vi "keccak.ip.fifo.control.vi"(10 "FIFO.inputs":T2, 11 "Reset":bool) -> (3 "FIFO.outputs":T1)   [LabVIEW 2021]
uses:
  Users/johns/OneDrive/Documents/LabVIEW Data/Untitled Project 2/CLIP/keccak.variables.ctl
  Users/johns/OneDrive/Documents/LabVIEW Data/Untitled Project 2/CLIP/keccak.states.ctl
  <vilib>/rvi/Emulation/niFpgaEmulationIsFPGAContextNoSignature.vi
  <vilib>/rvi/Emulation/niFpgaSctlEmulationGetInTimedLoop.vi
  <vilib>/rvi/errors/niFpgaSetErrorForExecOnDevCompSimple.vi
  <vilib>/rvi/eio/common/nirviEmuReportErrorAndStop.vi
  <vilib>/rvi/DataTransferAndStorage/Container/Common/niFpgaContainerGetUniqueNameForEmu.vi
  <vilib>/rvi/FIFO/Fifo_Resource/nirvififoEmulationSetSize.vi
  <vilib>/rvi/FIFO/Fifo_Resource/nirviFifoEmulationQueueMgr.vi
  <instcachedir>/0/nirviFifoEmulationQueueMgr_E5CAEC123FF24DC58D834DCA3CDAA9B5.lvgen/nirviFifoEmulationQueueMgr_E5CAEC123FF24DC58D834DCA3CDAA9B5_000.vi
  <vilib>/Utility/error.llb/Clear Errors.vi
  <vilib>/rvi/FIFO/Fifo_Resource/nirvififoEmulationCreateLock.vi
  <vilib>/rvi/Emulation/niFpgaProcessEmulError.vi
  <vilib>/rvi/FIFO/Fifo_Resource/nirvififoEmulationObtainLock.vi
  <vilib>/rvi/FIFO/Fifo_Resource/nirvififoEmulationReleaseLock.vi
  <vilib>/rvi/occurrence/nirviWaitOnOccurrenceBase.vi
  <vilib>/rvi/errors/nirviReportUnexpectedCaseInternalError.vi
  <vilib>/rvi/errors/nirviReportUnexpectedCaseInternalError (U32).vi
  <vilib>/rvi/FIFO/Fifo_Resource/nirvififoEmulationDetermineInputValidOut.vi
  <vilib>/rvi/DataTransferAndStorage/Container/XNode/niFpgaContainer.xnode
  <vilib>/rvi/FIFO/Fifo_Resource/nirvififoEmulationRead.vi
  <vilib>/rvi/FIFO/Fifo_Resource/nirvififoEmulationWrite.vi
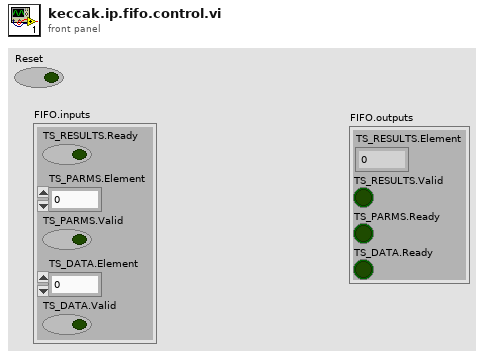
[diagram p1: front panel]
types:
  T1 = cluster{"TS_RESULTS.Element":u64, "TS_RESULTS.Valid":bool, "TS_PARMS.Ready":bool, "TS_DATA.Ready":bool}
  T2 = cluster{"TS_RESULTS.Ready":bool, "TS_PARMS.Element":u64, "TS_PARMS.Valid":bool, "TS_DATA.Element":u64, "TS_DATA.Valid":bool}
  T3 = typedef "keccak.variables.ctl" = cluster{"hash.input_size":u16, "hash.bits":u16, "state.next":T4, "state.after_next":T4, "read.i":u16, "read.block_i":u16, "hash.block_words":u16, "hash.block_size":u16, "keccak.i":u16, "state[25]":u64[], "HT_PARMS.Valid":bool, "HT_PARMS.Data":u64, "Read.HT_PARMS":bool, "HT_DATA.Valid":bool, "HT_DATA.Data":u64, "Read.HT_DATA":bool, "TH_RESULTS.Valid":bool, "TH_RESULTS.Data":u64, "TH_RESULTS.Ready":bool}
  T4 = typedef "keccak.states.ctl" = enum8{"Wait.for.Start", "Read.Blocks", "Read.Remainder", "Keccak", "Send.Result"}
  T5 = cluster{"Element":u64, bool, "Timed Out?":bool, "Ready for Input":bool}
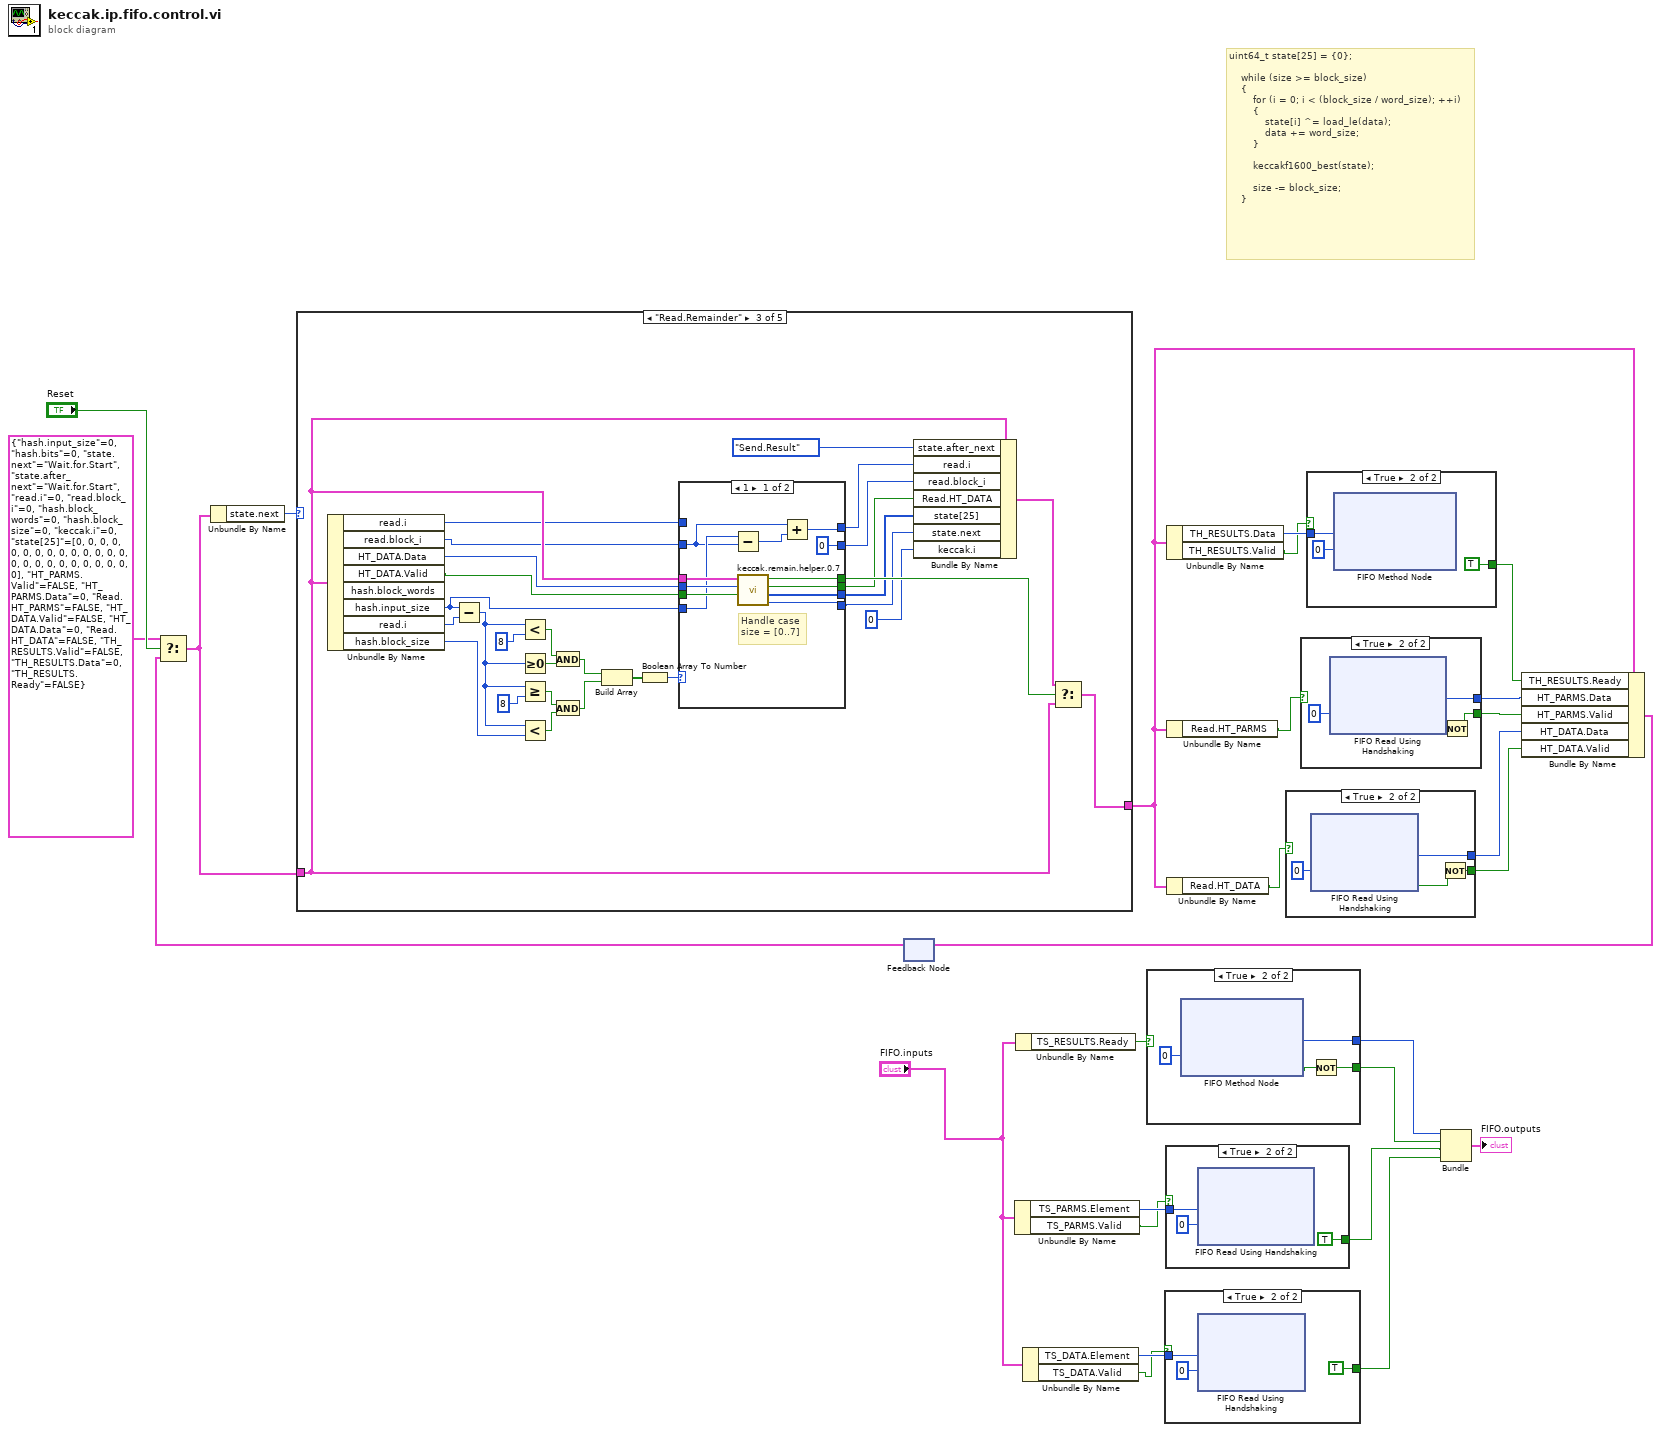
[diagram p0: block diagram]
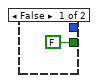
[diagram p2: hidden frame]
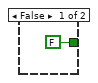
[diagram p3: hidden frame]
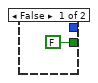
[diagram p4: hidden frame]
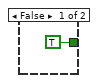
[diagram p5: hidden frame]
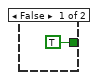
[diagram p6: hidden frame]
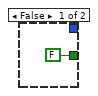
[diagram p7: hidden frame]
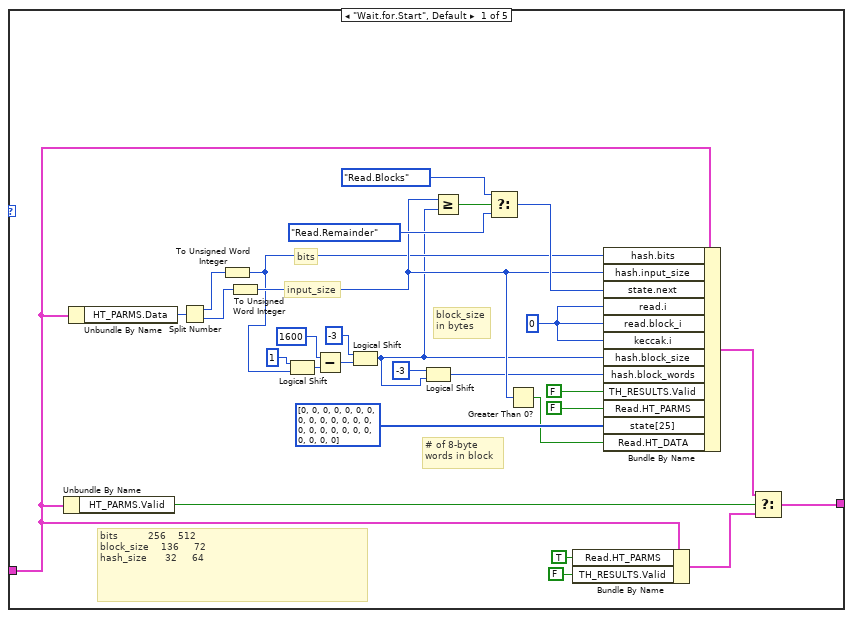
[diagram p8: hidden frame]
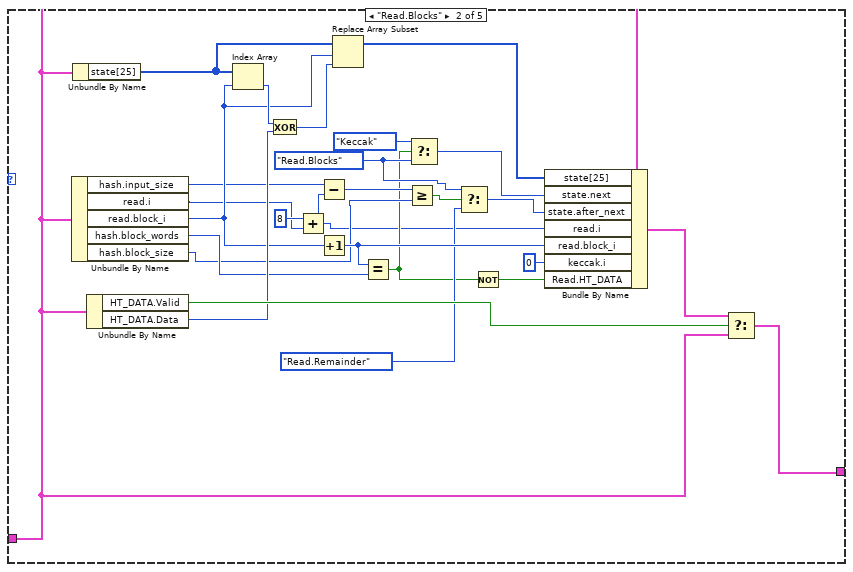
[diagram p9: hidden frame]
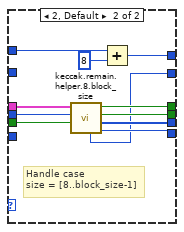
[diagram p10: hidden frame]
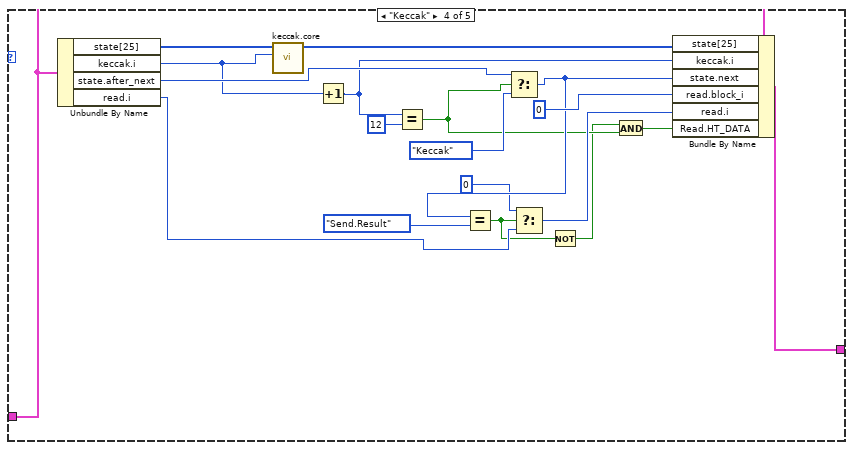
[diagram p11: hidden frame]
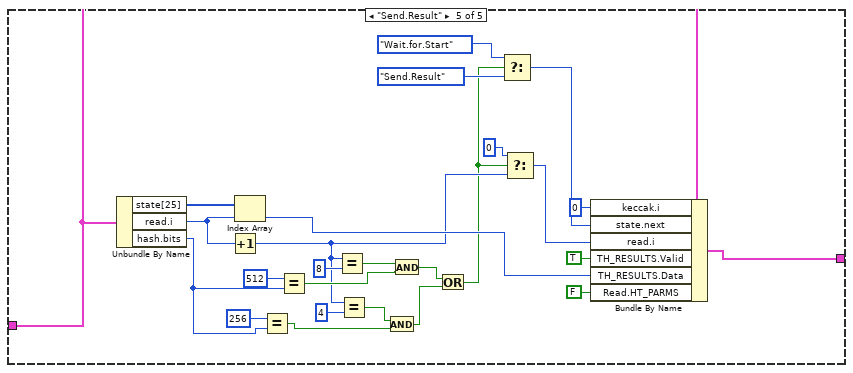
[diagram p12: hidden frame]
diagram:
  # "uint64_t state[25] = {0};\n\n    while (size >= block_size)\n    {\n        for (i = 0; i < (block_size / word_size); ++i)\n        {\n            state[i] ^= load_le(data);\n            data += word_size;\n        }\n\n        keccakf1600_best(state);\n\n        size -= block_size;\n    }"
  n1 = feedback #1() -> (w16:T3)  [unwired: 1 in]
  n2 = Select(t=T3 {"hash.input_size"=0, "hash.bits"=0, "state.next"=enum."Wait.for.Start", "state.after_next"=enum."Wait.for.Start", "read.i"=0, "read.block_i"=0, "hash.block_words"=0, "hash.block_size"=0, "keccak.i"=0, "state[25]"=[0, 0, 0, 0, 0, 0, 0, 0, 0, 0, 0, 0, 0, 0, 0, 0, 0, 0, 0, 0, 0, 0, 0, 0, 0], "HT_PARMS.Valid"=FALSE, "HT_PARMS.Data"=0, "Read.HT_PARMS"=FALSE, "HT_DATA.Valid"=FALSE, "HT_DATA.Data"=0, "Read.HT_DATA"=FALSE, "TH_RESULTS.Valid"=FALSE, "TH_RESULTS.Data"=0, "TH_RESULTS.Ready"=FALSE} ("Variables"), s="Reset", f=w16) -> (s? t:f=w15:T3)
  n3 = Unbundle By Name(w15) -> ("state.next"=w27:T4)
  n4 = case shown="\"Read.Remainder\"" w27 {
    tunnel: [w52 w82 w109 w152 w180] -> w22
    tunnel: w15 -> [w47 w81 w105 w153 w179]
    frame "Wait.for.Start", Default {
      w37 = u16 0 ("read.i")
      # "# of 8-byte\nwords in block"
      # "block_size\nin bytes"
      # "bits"
      # "input_size"
      # "bits          256    512\nblock_size    136     72\nhash_size      32     64"
      n5 = Unbundle By Name(w47) -> ("HT_PARMS.Valid"=w51:bool)
      n6 = Unbundle By Name(w47) -> ("HT_PARMS.Data"=w56:u64)
      n7 = Split Number(x=w56) -> (hi(x)=w55:u32, lo(x)=w54:u32)
      n8 = To Unsigned Word Integer(number=w55) -> (unsigned 16bit integer=w29:u16)
      n9 = To Unsigned Word Integer(number=w54) -> (unsigned 16bit integer=w39:u16)
      n10 = Logical Shift(y=i16 1, x=w29) -> (x << y=w34:u16)
      n11 = Subtract(x=u16 1600, y=w34) -> (x-y=w33:u16)
      n12 = Logical Shift(y=i16 -3, x=w33) -> (x << y=w28:u16)
      n13 = Logical Shift(y=i16 -3, x=w28) -> (x << y=w30:u16)
      n14 = Greater Or Equal?(x=w39, y=w28) -> (x >= y?=w43:bool)
      n15 = Select(t=keccak.states."Read.Blocks" ("state.next"), s=w43, f=keccak.states."Read.Remainder" ("state.next")) -> (s? t:f=w41:T4)
      n16 = Greater Than 0?(x=w39) -> (x > 0?=w38:bool)
      n17 = Bundle By Name(cluster=w47, "Read.HT_PARMS"=TRUE, "TH_RESULTS.Valid"=FALSE) -> (w48:T3)
      n18 = Bundle By Name(cluster=w47, "hash.bits"=w29, "hash.input_size"=w39, "state.next"=w41, "read.i"=w37, "read.block_i"=w37, "keccak.i"=w37, "hash.block_size"=w28, "hash.block_words"=w30, "TH_RESULTS.Valid"=FALSE, "Read.HT_PARMS"=FALSE, "state[25]"=u64[] [0, 0, 0, 0, 0, 0, 0, 0, 0, 0, 0, 0, 0, 0, 0, 0, 0, 0, 0, 0, 0, 0, 0, 0, 0] ("state[24]"), "Read.HT_DATA"=w38) -> (w53:T3)
      n19 = Select(t=w53, s=w51, f=w48) -> (s? t:f=w52:T3)
    }
    frame "Read.Blocks" {
      w62 = keccak.states."Read.Blocks" ("state.next")
      n20 = Unbundle By Name(w81) -> ("hash.input_size"=w67:u16, "read.i"=w66:u16, "read.block_i"=w75:u16, "hash.block_words"=w71:u16, "hash.block_size"=w63:u16)
      n21 = Unbundle By Name(w81) -> ("state[25]"=w79:u64[])
      n22 = Unbundle By Name(w81) -> ("HT_DATA.Valid"=w80:bool, "HT_DATA.Data"=w76:u64)
      n23 = Index Array(array=w79, index=w75) -> (element=w78:u64)
      n24 = Exclusive Or(1:w76, 2:w78) -> (0:w77:u64)
      n25 = Add(x=u16 8, y=w66) -> (x+y=w57:u16)
      n26 = Subtract(x=w67, y=w57) -> (x-y=w64:u16)
      n27 = Increment(x=w75) -> (x+1=w72:u16)
      n28 = Replace Array Subset(array=w79, new element=w77, index=w75) -> (w68:u64[])
      n29 = Equal?(x=w72, y=w71) -> (x = y?=w59:bool)
      n30 = Greater Or Equal?(x=w64, y=w63) -> (x >= y?=w65:bool)
      n31 = Select(t=keccak.states."Keccak" ("state.next"), s=w59, f=w62) -> (s? t:f=w73:T4)
      n32 = Select(t=w62, s=w65, f=keccak.states."Read.Remainder" ("state.next")) -> (s? t:f=w69:T4)
      n33 = Not(x=w59) -> (.not. x?=w58:bool)
      n34 = Bundle By Name(cluster=w81, "state[25]"=w68, "state.next"=w73, "state.after_next"=w69, "read.i"=w57, "read.block_i"=w72, "keccak.i"=u16 0, "Read.HT_DATA"=w58) -> (w83:T3)
      n35 = Select(t=w83, s=w80, f=w81) -> (s? t:f=w82:T3)
    }
    frame "Read.Remainder" {
      n36 = Unbundle By Name(w105) -> ("read.i"=w89:u16, "read.block_i"=w90:u16, "HT_DATA.Data"=w104:u64, "HT_DATA.Valid"=w103:bool, "hash.input_size"=w88:u16, "read.i"=w112:u16, "hash.block_size"=w92:u16)  [unwired: 1 out]
      n37 = Subtract(x=w88, y=w112) -> (x-y=w93:u16)
      n38 = Less?(x=w93, y=u16 8) -> (x < y?=w101:bool)
      n39 = Greater Or Equal To 0?(x=w93) -> (x >= 0?=w102:bool)
      n40 = Greater Or Equal?(x=w93, y=u16 8) -> (x >= y?=w96:bool)
      n41 = Less?(x=w93, y=w92) -> (x < y?=w91:bool)
      n42 = And(x=w101, y=w102) -> (x .and. y?=w98:bool)
      n43 = And(x=w96, y=w91) -> (x .and. y?=w95:bool)
      n44 = Build Array(w98, w95) -> (w99:bool[])
      n45 = Boolean Array To Number(Boolean array=w99) -> (number=w97:u8)
      n46 = case shown="1" w97 {
        tunnel: [w124 w131] -> w108
        tunnel: [w123 w132] -> w107
        tunnel: [w122 w130] -> w106
        tunnel: w105 -> [w121 w135]
        tunnel: w104 -> [w120 w134]
        tunnel: w103 -> [w119 w133]
        tunnel: [w118 w126] -> w87
        tunnel: w90 -> [w115 _]
        tunnel: [u16 0 w125] -> w85
        tunnel: [w114 w128] -> w84
        tunnel: w89 -> [_ w127]
        tunnel: w88 -> [w116 _]
        frame 1 {
          # "Handle case\nsize = [0..7]"
          n47 = Subtract(x=w116, y=w115) -> (x-y=w113:u16)
          n48 = call "keccak.remain.helper.0.7.vi"("HT_DATA.Valid"=w119, "HT_DATA.Data"=w120, "Variables"=w121) -> ("state.next"=w118:T4, "state[25] out"=w122:u64[], "Continue?"=w123:bool, "Valid"=w124:bool)  [unwired: 5 in]
          n49 = Add(x=w115, y=w113) -> (x+y=w114:u16)
        }
        frame 2, Default {
          # "Handle case\nsize = [8..block_size-1]"
          n50 = call "keccak.remain.helper.8.block_size.vi"("HT_DATA.Valid"=w133, "HT_DATA.Data"=w134, "Variables"=w135) -> ("state.next"=w126:T4, "state[25] out"=w130:u64[], "Continue?"=w132:bool, "Valid"=w131:bool, "read.block_i"=w125:u16)  [unwired: 4 in]
          n51 = Add(x=w127, y=u16 8) -> (x+y=w128:u16)
        }
      }
      n52 = Bundle By Name(cluster=w105, "state.after_next"=keccak.states."Send.Result" ("state.next"), "read.i"=w84, "read.block_i"=w85, "Read.HT_DATA"=w107, "state[25]"=w106, "state.next"=w87, "keccak.i"=u16 0) -> (w110:T3)
      n53 = Select(t=w110, s=w108, f=w105) -> (s? t:f=w109:T3)
    }
    frame "Keccak" {
      n54 = Unbundle By Name(w153) -> ("state[25]"=w154:u64[], "keccak.i"=w146:u16, "state.after_next"=w148:T4, "read.i"=w143:u16)
      n55 = call "keccak.core.vi"("keccak.i"=w146, "state[25]"=w154) -> ("state[25].out"=w151:u64[])  [unwired: 9 in]
      n56 = Increment(x=w146) -> (x+1=w147:u16)
      n57 = Equal?(x=w147, y=u16 12) -> (x = y?=w139:bool)
      n58 = Select(t=w148, s=w139, f=keccak.states."Keccak" ("state.next")) -> (s? t:f=w142:T4)
      n59 = Equal?(x=w142, y=keccak.states."Send.Result" ("state.next")) -> (x = y?=w137:bool)
      n60 = Select(t=u16 0, s=w137, f=w143) -> (s? t:f=w144:u16)
      n61 = Not(x=w137) -> (.not. x?=w136:bool)
      n62 = And(x=w136, y=w139) -> (x .and. y?=w138:bool)
      n63 = Bundle By Name(cluster=w153, "state[25]"=w151, "keccak.i"=w147, "state.next"=w142, "read.block_i"=u16 0 ("read.i"), "read.i"=w144, "Read.HT_DATA"=w138) -> (w152:T3)
    }
    frame "Send.Result" {
      n64 = Unbundle By Name(w179) -> ("state[25]"=w178:u64[], "read.i"=w177:u16, "hash.bits"=w167:u16)
      n65 = Increment(x=w177) -> (x+1=w160:u16)
      n66 = Index Array(array=w178, index=w177) -> (element=w168:u64)
      n67 = Equal?(x=u16 256, y=w167) -> (x = y?=w164:bool)
      n68 = Equal?(x=u16 512, y=w167) -> (x = y?=w173:bool)
      n69 = Equal?(x=w160, y=u16 8) -> (x = y?=w174:bool)
      n70 = Equal?(x=w160, y=u16 4) -> (x = y?=w163:bool)
      n71 = And(x=w163, y=w164) -> (x .and. y?=w162:bool)
      n72 = And(x=w174, y=w173) -> (x .and. y?=w161:bool)
      n73 = Or(x=w161, y=w162) -> (x .or. y?=w158:bool)
      n74 = Select(t=keccak.states."Wait.for.Start" ("state.next"), s=w158, f=keccak.states."Send.Result" ("state.next")) -> (s? t:f=w170:T4)
      n75 = Select(t=u16 0, s=w158, f=w160) -> (s? t:f=w159:u16)
      n76 = Bundle By Name(cluster=w179, "keccak.i"=u16 0, "state.next"=w170, "read.i"=w159, "TH_RESULTS.Valid"=TRUE, "TH_RESULTS.Data"=w168, "Read.HT_PARMS"=FALSE) -> (w180:T3)
    }
  }
  n77 = Unbundle By Name("FIFO.inputs") -> ("TS_PARMS.Element"=w14:u64, "TS_PARMS.Valid"=w5:bool)
  n78 = Unbundle By Name("FIFO.inputs") -> ("TS_RESULTS.Ready"=w7:bool)
  n79 = Unbundle By Name("FIFO.inputs") -> ("TS_DATA.Element"=w13:u64, "TS_DATA.Valid"=w4:bool)
  n80 = case shown="True" w7 {
    tunnel: [_ w185] -> w11
    tunnel: [FALSE w182] -> w6
    frame False {
    }
    frame True {
      n81 = xnode ("FIFO Method Node")("Timeout"=0) -> ("Element"=w185:u64, "Timed Out?"=w183:bool)  [unwired: 1 in, 1 out]
      n82 = Not(x=w183) -> (.not. x?=w182:bool)
    }
  }
  n83 = case shown="True" w4 {
    tunnel: w13 -> [_ w189]
    tunnel: [TRUE ("Ready for Input") TRUE ("Ready for Input")] -> w9
    frame False {
    }
    frame True {
      n84 = xnode ("FIFO Read Using Handshaking")("Element"=w189, "Timeout"=0) -> ()  [unwired: 1 in, 2 out]
    }
  }
  n85 = case shown="True" w5 {
    tunnel: w14 -> [_ w193]
    tunnel: [TRUE ("Timed Out?") TRUE ("Timed Out?")] -> w10
    frame False {
    }
    frame True {
      n86 = xnode ("FIFO Read Using Handshaking")("Element"=w193, "Timeout"=0) -> ()  [unwired: 1 in, 2 out]
    }
  }
  n87 = Unbundle By Name(w22) -> ("TH_RESULTS.Data"=w21:u64, "TH_RESULTS.Valid"=w2:bool)
  n88 = Unbundle By Name(w22) -> ("Read.HT_PARMS"=w1:bool)
  n89 = Unbundle By Name(w22) -> ("Read.HT_DATA"=w3:bool)
  n90 = case shown="True" w3 {
    tunnel: [FALSE w196] -> w24
    tunnel: [_ w198] -> w23
    frame False {
    }
    frame True {
      n91 = xnode ("FIFO Read Using Handshaking")("Timeout"=0) -> ("Element"=w198:u64, "Timed Out?"=w197:bool)  [unwired: 1 in, 1 out]
      n92 = Not(x=w197) -> (.not. x?=w196:bool)
    }
  }
  n93 = case shown="True" w1 {
    tunnel: [FALSE w200] -> w26
    tunnel: [_ w203] -> w25
    frame False {
    }
    frame True {
      n94 = xnode ("FIFO Read Using Handshaking")("Timeout"=0) -> ("Element"=w203:u64, "Timed Out?"=w201:bool)  [unwired: 1 in, 1 out]
      n95 = Not(x=w201) -> (.not. x?=w200:bool)
    }
  }
  n96 = case shown="True" w2 {
    tunnel: w21 -> [_ w207]
    tunnel: [FALSE TRUE] -> w20
    frame False {
    }
    frame True {
      n97 = xnode ("FIFO Method Node")("Element"=w207, "Timeout"=0) -> ()  [unwired: 1 in, 2 out]
    }
  }
  n98 = Bundle("Element"=w11, w6, "Timed Out?"=w10, "Ready for Input"=w9) -> (→"FIFO.outputs":T5)  [unwired: 1 in]
  n99 = Bundle By Name(cluster=w22, "TH_RESULTS.Ready"=w20, "HT_PARMS.Data"=w25, "HT_PARMS.Valid"=w26, "HT_DATA.Data"=w23, "HT_DATA.Valid"=w24) -> (w19:T3)
  n100 = feedback-in #1(w19) -> ()
